vi "test_riccat_02i.vi"() -> (3 "All Tests Passed":bool)   [LabVIEW 2019]
uses:
  <vilib>/Analysis/Matrix/Datatypes/RealMatrix.ctl
  <vilib>/Analysis/7linalg.llb/Real Transpose Matrix.vi
  <vilib>/Analysis/baseanly.llb/Real A x B.vi
  <vilib>/Analysis/Matrix/Numeric/Subtract/Subtract - RM,RM.vi
  <vilib>/Analysis/Matrix/Numeric/Add/Add - RM,RM.vi
  <vilib>/Analysis/baseanly.llb/Real Inverse Matrix.vi
  <vilib>/Analysis/Matrix/Numeric/Absolute Value/Absolute Value - RM.vi
  <vilib>/Rock Robotics/WPI/ThirdParty/JAS_Junk/TrajLib/Trajectory_Library.lvlib
  <vilib>/Analysis/NI_AALPro.lvlib
  <vilib>/Analysis/NI_AALBase.lvlib
  <vilib>/Analysis/Matrix/NI_Matrix.lvlib
panel:
  out "Error":bool
  out "Iterations":i32
  out "Elapsed \nTime MS":dbl
  out "Err 4":i32
  out "Err 3":i32
  out "Err 2":i32
  out "Err 1":i32
  out "Err 9":i32
  out "ZERO":T1
  out "X  Answer":T1
  in  "R":T1=[[0.3]]
  in  "Q":T1=[[1.0, 0.0], [0.0, 0.0]]
  in  "B":T1=[[0.0], [1.0]]
  in  "A":T1=[[1.0, 1.0], [0.0, 1.0]]
  # "// ------------------------------------------------------------\n  // Test 2: invertible A"
  # "A2 << \n             1, 1, \n              0, 1;"
  # "B2 << \n        0, \n        1;"
  # "Solution weight ??"
  # "Q2 << \n         1, 0, \n         0, 0;"
  # "Example G2"
  # "Cost ??"
  # "R2 << 0.3;"
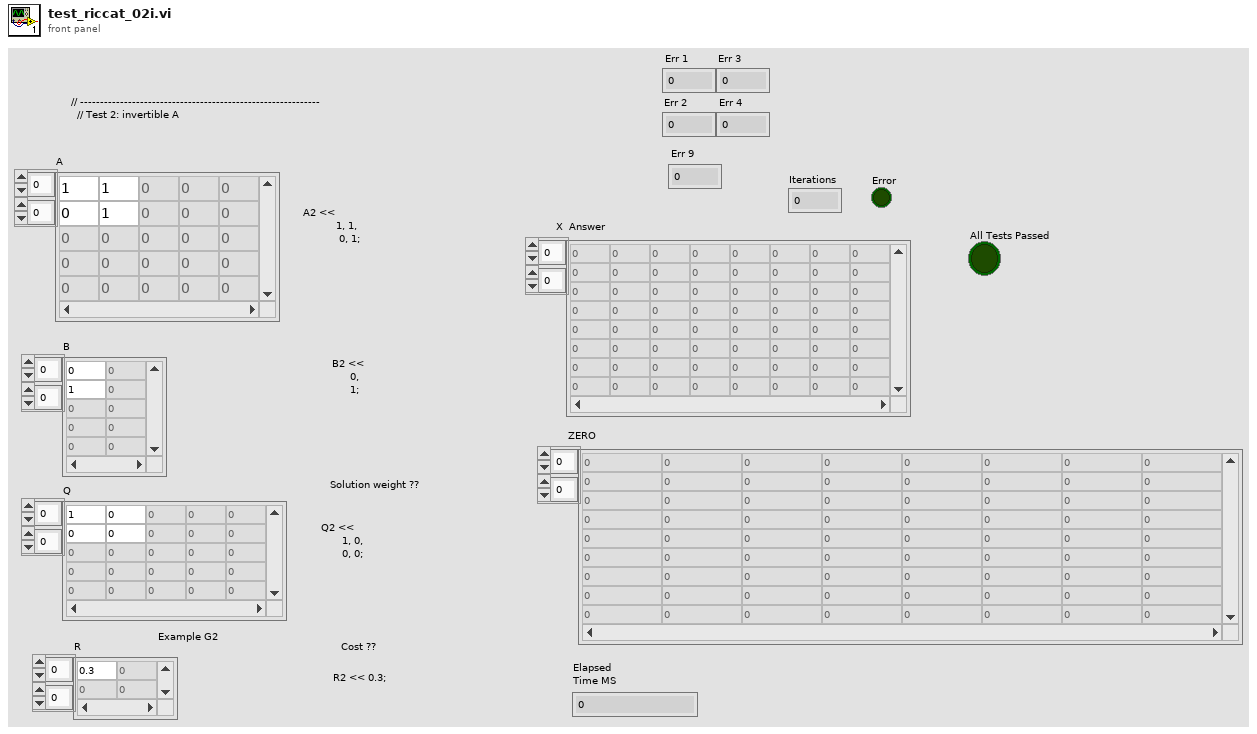
[diagram p1: front panel]
types:
  T1 = typedef "NI_Matrix.lvlib/RealMatrix.ctl" = dbl[][]
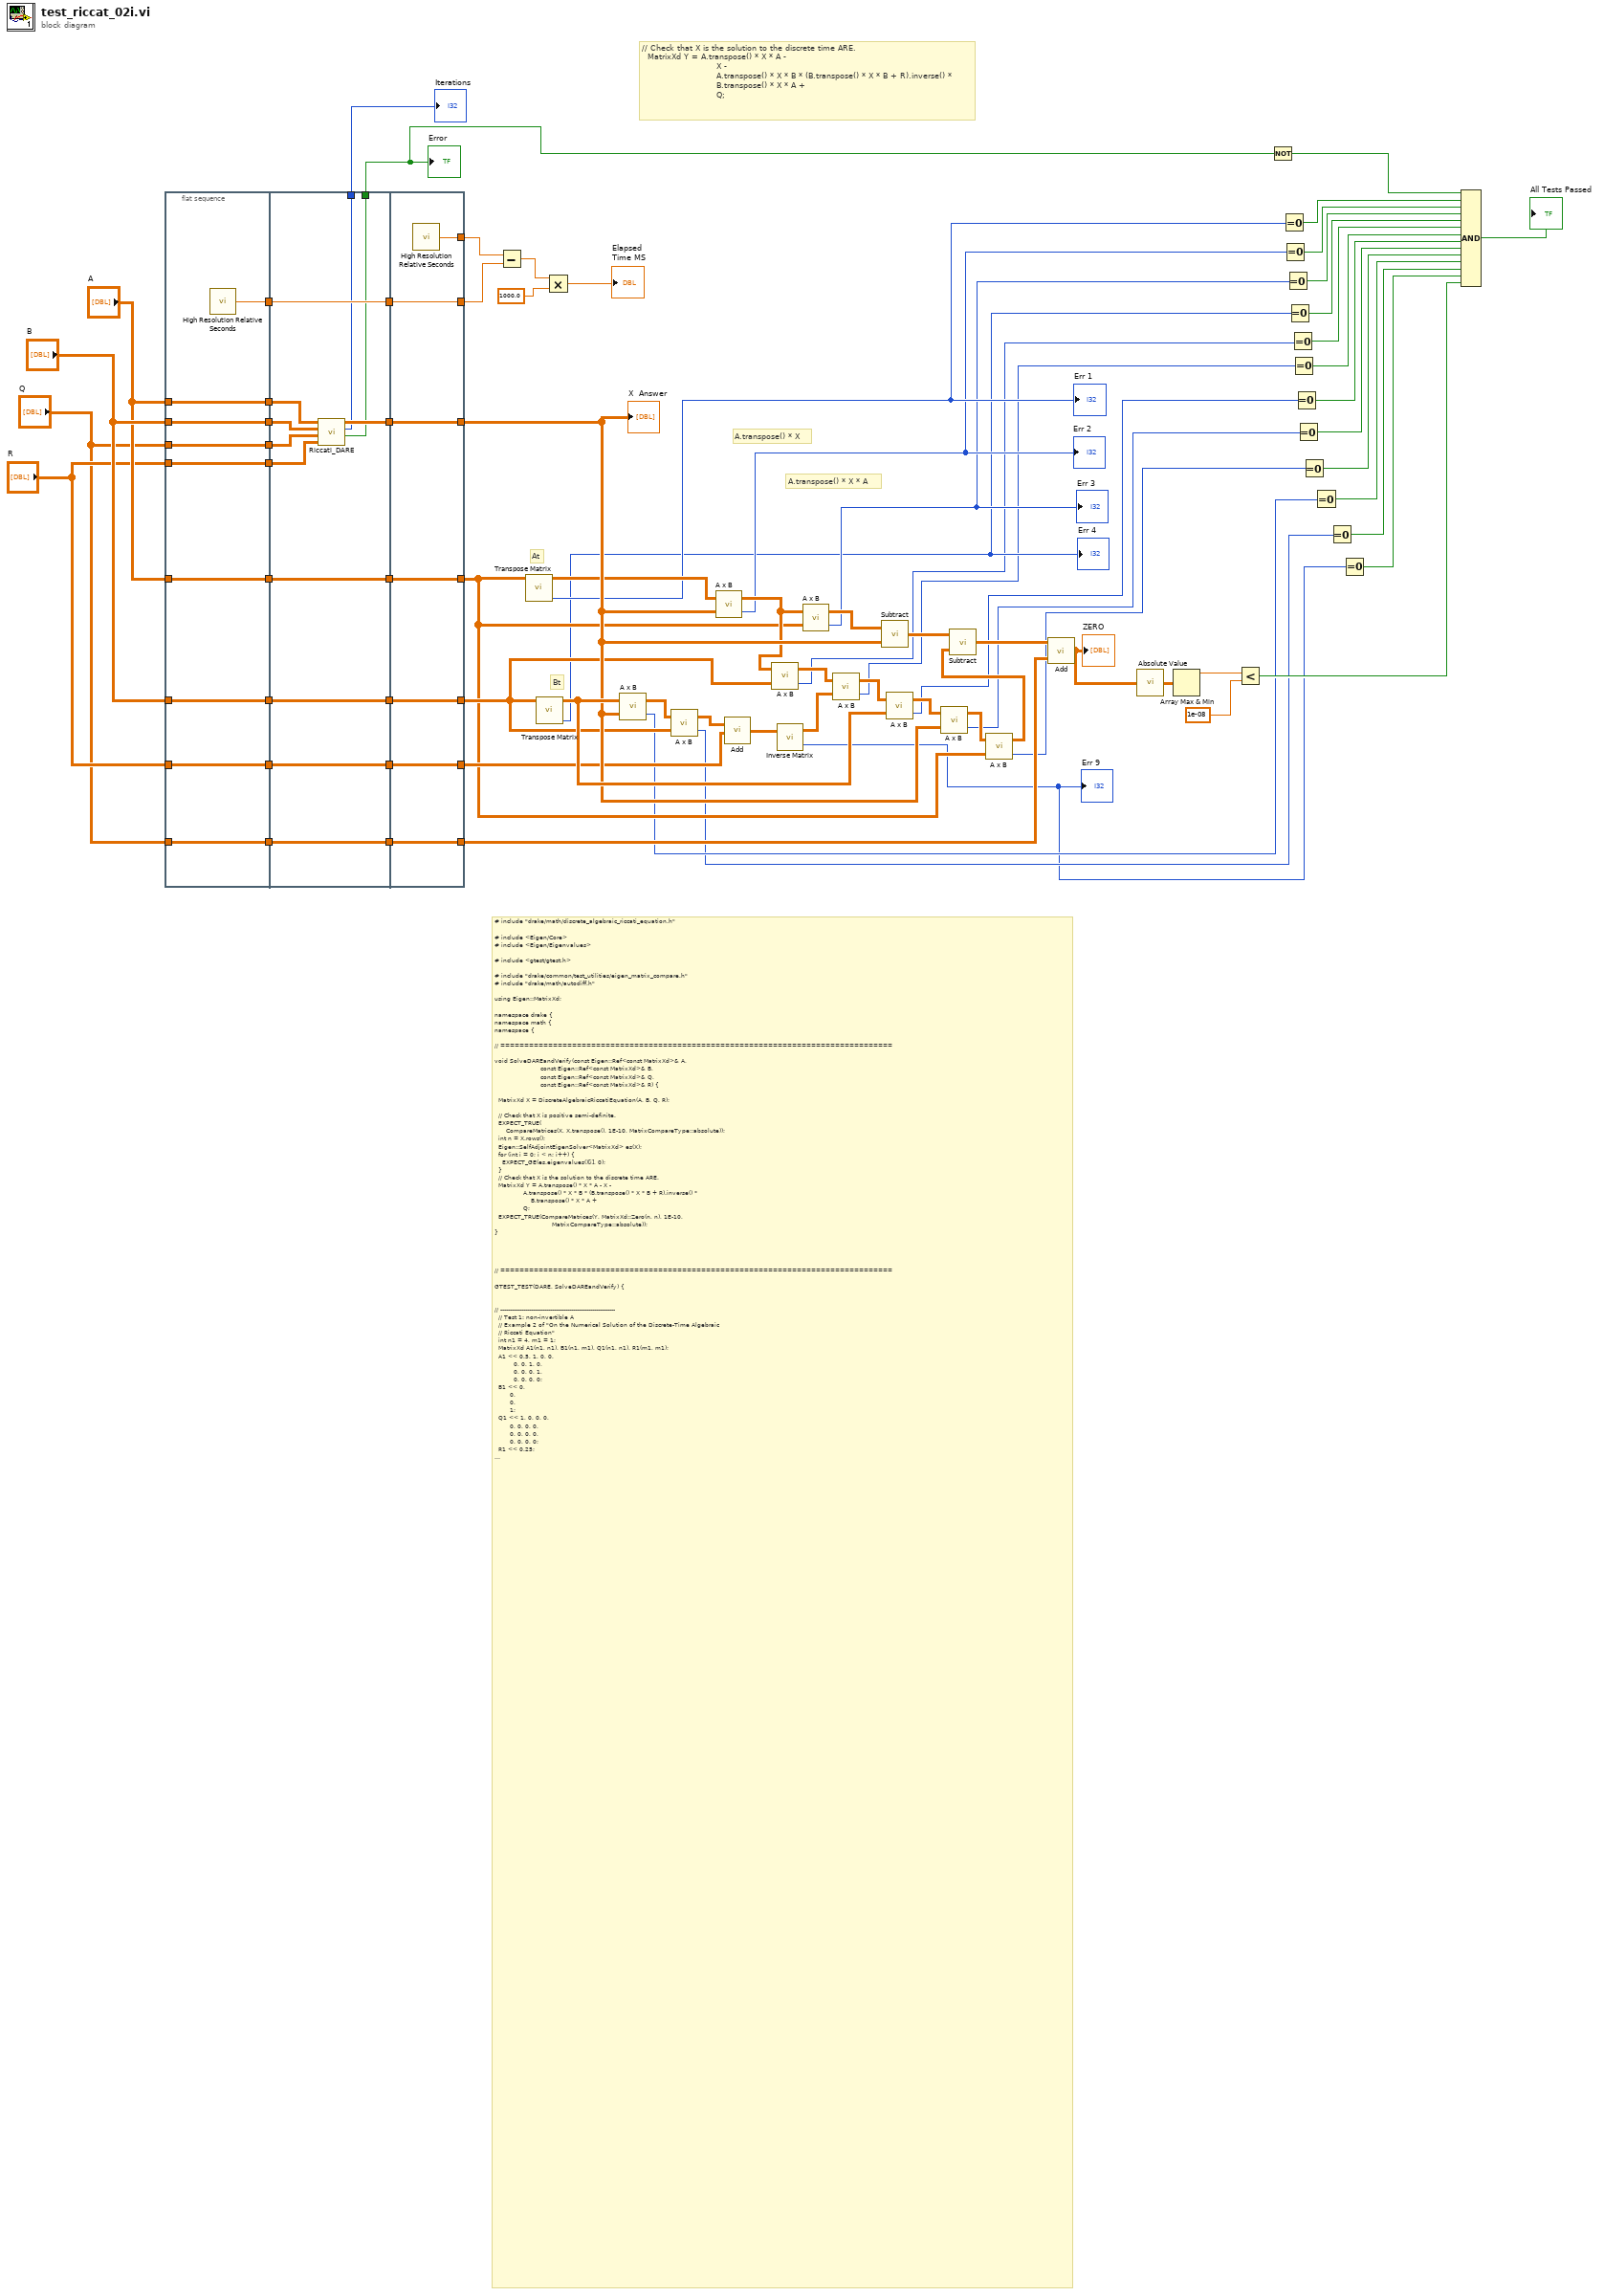
[diagram p0: block diagram]
diagram:
  # "A.transpose() * X"
  # "A.transpose() * X * A"
  # "Bt"
  # "At"
  # "// Check that X is the solution to the discrete time ARE.\n  MatrixXd Y = A.transpose() * X * A - \n                          X -\n                          A.transpose() * X * B * (B.transpose() * X * B + R).inverse() *\n                          B.transpose() * X * A +\n                          Q;"
  # "# include \"drake/math/discrete_algebraic_riccati_equation.h\"\n\n# include <Eigen/Core>\n# include <Eigen/Eigenvalues>\n\n# include <gtest/gtest.h>\n\n# include \"drake/common/test_utilities/eigen_matrix_compare.h\"\n# include \"drake/math/autodiff.h\"\n\nusing Eigen::MatrixXd;\n\nnamespace drake {\nnamespace math {\nnamespace {\n\n// ==================================================================================\n\nvoid SolveDAREandVerify(const Eigen::Ref<const MatrixXd>& A,\n                        const Eigen::Ref<const MatrixXd>& B,\n                        const Eigen::Ref<const MatrixXd>& Q,\n                        const Eigen::Ref<const MatrixXd>& R) {\n\n  MatrixXd X = DiscreteAlgebraicRiccatiEquation(A, B, Q, R);\n\n  // Check that X is positive semi-definite.\n  EXPECT_TRUE(\n      CompareMatrices(X, X.transpose(), 1E-10, MatrixCompareType::absolute));\n  int n = X.rows();\n  Eigen::SelfAdjointEigenSolver<MatrixXd> es(X);\n  for (int i = 0; i < n; i++) {\n    EXPECT_GE(es.eigenvalues()[i], 0);\n  }\n  // Check that X is the solution to the discrete time ARE.\n  MatrixXd Y = A.transpose() * X * A - X -\n               A.transpose() * X * B * (B.transpose() * X * B + R).inverse() *\n                   B.transpose() * X * A +\n               Q;\n  EXPECT_TRUE(CompareMatrices(Y, MatrixXd::Zero(n, n), 1E-10,\n                              MatrixCompareType::absolute));\n}\n\n\n\n\n// ==================================================================================\n\nGTEST_TEST(DARE, SolveDAREandVerify) {\n\n\n// ------------------------------------------------------------\n  // Test 1: non-invertible A\n  // Example 2 of \"On the Numerical Solution of the Discrete-Time Algebraic\n  // Riccati Equation\"\n  int n1 = 4, m1 = 1;\n  MatrixXd A1(n1, n1), B1(n1, m1), Q1(n1, n1), R1(m1, m1);\n  A1 << 0.5, 1, 0, 0, \n          0, 0, 1, 0, \n          0, 0, 0, 1, \n          0, 0, 0, 0;\n  B1 << 0, \n        0, \n        0, \n        1;\n  Q1 << 1, 0, 0, 0, \n        0, 0, 0, 0, \n        0, 0, 0, 0, \n        0, 0, 0, 0;\n  R1 << 0.25;\n  SolveDAREandVerify(A1, B1, Q1, R1);\n// ------------------------------------------------------------\n  // Test 2: invertible A\n  int n2 = 2, m2 = 1;\n  MatrixXd A2(n2, n2), B2(n2, m2), Q2(n2, n2), R2(m2, m2);\n  A2 << 1, 1, 0, 1;\n  B2 << 0, 1;\n  Q2 << 1, 0, 0, 0;\n  R2 << 0.3;\n  SolveDAREandVerify(A2, B2, Q2, R2);\n\n// ------------------------------------------------------------\n  // Test 3: the first generalized eigenvalue of (S,T) is stable\n  int n3 = 2, m3 = 1;\n  MatrixXd A3(n3, n3), B3(n3, m3), Q3(n3, n3), R3(m3, m3);\n  A3 << 0, 1, 0, 0;\n  B3 << 0, 1;\n  Q3 << 1, 0, 0, 1;\n  R3 << 1;\n  SolveDAREandVerify(A3, B3, Q3, R3);\n\n// ------------------------------------------------------------\n  // Test 4: A = B = Q = R = I_2 (2-by-2 identity matrix)\n  int n4 = 2, m4 = 2;\n  MatrixXd A4(n4, n4), B4(n4, m4), Q4(n4, n4), R4(m4, m4);\n  A4 << 1, 0, 0, 1;\n  B4 << 1, 0, 0, 1;\n  Q4 << 1, 0, 0, 1;\n  R4 << 1, 0, 0, 1;\n  SolveDAREandVerify(A4, B4, Q4, R4);\n\n// ------------------------------------------------------------\n}\n}  // namespace\n}  // namespace math\n}  // namespace drake"
  n1 = flat-sequence {
    tunnel: "B" -> [w81]
    tunnel: "A" -> [w82]
    tunnel: "B" -> [w83]
    tunnel: "Q" -> [w84]
    tunnel: "A" -> [w85]
    tunnel: "R" -> [w86]
    tunnel: [w86] -> w61
    tunnel: [w85] -> w60
    tunnel: [w84] -> w59
    tunnel: [w83] -> w58
    tunnel: [w82] -> w57
    tunnel: [w81] -> w56
    tunnel: "R" -> [w80]
    tunnel: [w80] -> w48
    tunnel: "Q" -> [w79]
    tunnel: [w79] -> w45
    tunnel: [w78] -> w38
    tunnel: w61 -> [w98]
    tunnel: w60 -> [w96]
    tunnel: w59 -> [w95]
    tunnel: w58 -> [w94]
    tunnel: w57 -> [w93]
    tunnel: w56 -> [w92]
    tunnel: [w97] -> w55
    tunnel: [w93] -> w54
    tunnel: [w92] -> w53
    tunnel: [w91] -> w49
    tunnel: w48 -> [w91]
    tunnel: w45 -> [w90]
    tunnel: [w90] -> w44
    tunnel: [w89] -> w39
    tunnel: w38 -> [w89]
    tunnel: [w88] -> w34
    tunnel: [w87] -> w18
    tunnel: [w103] -> w51
    tunnel: [w104] -> w33
    tunnel: [w105] -> w69
    tunnel: w55 -> [w105]
    tunnel: w54 -> [w104]
    tunnel: w53 -> [w103]
    tunnel: [w102] -> w46
    tunnel: w49 -> [w102]
    tunnel: [w101] -> w42
    tunnel: w44 -> [w101]
    tunnel: [w100] -> w41
    tunnel: [w99] -> w40
    tunnel: w39 -> [w99]
    frame #0 {
      n2 = call <vilib>:"High Resolution Relative Seconds.vi"() -> ("relative seconds"=w78:dbl)
    }
    frame #1 {
      n3 = call <vilib>:"Riccati_DARE.vi"("R"=w98, "Q"=w95, "B"=w94, "A"=w96) -> ("Error"=w87:bool, "Iterations"=w88:i32, "Answer"=w97:T1)  [unwired: 5 in]
    }
    frame #2 {
      n4 = call <vilib>:"High Resolution Relative Seconds.vi"() -> ("relative seconds"=w100:dbl)
    }
  }
  n5 = Subtract(x=w41, y=w40) -> (x-y=w37:dbl)
  n6 = call-poly <vilib>:"Transpose Matrix.vi"("Input Matrix"=w33) -> ("error"=w17:i32, "Matrix Transpose"=w62:T1)  [unwired: 9 in]
  "Err 1" <- w17
  n7 = call-poly <vilib>:"Transpose Matrix.vi"("Input Matrix"=w51) -> ("error"=w14:i32, "Matrix Transpose"=w71:T1)  [unwired: 9 in]
  "Err 4" <- w14
  n8 = Multiply(x=w37, y=1000.0) -> (x*y=→"Elapsed \nTime MS":dbl)
  n9 = call-poly <vilib>:"A x B.vi"("B"=w69, "A"=w71) -> ("error"=w3:i32, "A x B"=w76:T1)
  n10 = call-poly <vilib>:"A x B.vi"("B"=w51, "A"=w76) -> ("error"=w2:i32, "A x B"=w75:T1)
  n11 = call-poly <vilib>:"A x B.vi"("B"=w69, "A"=w62) -> ("error"=w16:i32, "A x B"=w64:T1)
  "Err 2" <- w16
  n12 = call-poly <vilib>:"Add.vi"("Real Matrix B"=w46, "Real Matrix A"=w75) -> ("A + B"=w74:T1)
  n13 = call-poly <vilib>:"A x B.vi"("B"=w51, "A"=w64) -> ("error"=w8:i32, "A x B"=w63:T1)
  n14 = call-poly <vilib>:"Inverse Matrix.vi"("Input Matrix"=w74) -> ("error"=w1:i32, "Inverse Matrix"=w73:T1)  [unwired: 1 in]
  "Err 9" <- w1
  n15 = call-poly <vilib>:"A x B.vi"("B"=w33, "A"=w64) -> ("error"=w15:i32, "A x B"=w77:T1)
  "Err 3" <- w15
  n16 = call-poly <vilib>:"A x B.vi"("B"=w73, "A"=w63) -> ("error"=w7:i32, "A x B"=w72:T1)
  n17 = call-poly <vilib>:"Subtract.vi"("Real Matrix B"=w69, "Real Matrix A"=w77) -> ("A - B"=w67:T1)
  n18 = call-poly <vilib>:"A x B.vi"("B"=w71, "A"=w72) -> ("error"=w6:i32, "A x B"=w70:T1)
  n19 = call-poly <vilib>:"A x B.vi"("B"=w69, "A"=w70) -> ("error"=w5:i32, "A x B"=w68:T1)
  n20 = call-poly <vilib>:"A x B.vi"("B"=w33, "A"=w68) -> ("error"=w4:i32, "A x B"=w66:T1)
  n21 = call-poly <vilib>:"Subtract.vi"("Real Matrix B"=w66, "Real Matrix A"=w67) -> ("A - B"=w65:T1)
  n22 = call-poly <vilib>:"Add.vi"("Real Matrix B"=w42, "Real Matrix A"=w65) -> ("A + B"=w13:T1)
  "ZERO" <- w13
  n23 = call-poly <vilib>:"Absolute Value.vi"("Real Matrix A"=w13) -> ("|A|"=w12:T1)
  n24 = Array Max & Min(array=w12) -> (max value=w11:dbl)  [unwired: 3 out]
  n25 = Less?(x=w11, y=1e-08) -> (x < y?=w9:bool)
  n26 = Not(x=w18) -> (.not. x?=w19:bool)
  n27 = Equal To 0?(x=w17) -> (x = 0?=w31:bool)
  n28 = Equal To 0?(x=w16) -> (x = 0?=w30:bool)
  n29 = Equal To 0?(x=w15) -> (x = 0?=w29:bool)
  n30 = Equal To 0?(x=w14) -> (x = 0?=w28:bool)
  n31 = Equal To 0?(x=w8) -> (x = 0?=w27:bool)
  n32 = Equal To 0?(x=w7) -> (x = 0?=w26:bool)
  n33 = Equal To 0?(x=w6) -> (x = 0?=w25:bool)
  n34 = Equal To 0?(x=w5) -> (x = 0?=w24:bool)
  n35 = Equal To 0?(x=w4) -> (x = 0?=w23:bool)
  n36 = Equal To 0?(x=w3) -> (x = 0?=w22:bool)
  n37 = Equal To 0?(x=w2) -> (x = 0?=w21:bool)
  n38 = Equal To 0?(x=w1) -> (x = 0?=w20:bool)
  n39 = Compound Arithmetic op=AND(w19, w31, w30, w29, w28, w27, w26, w25, w24, w23, w22, w21, w20, w9) -> (→"All Tests Passed":bool)
  "X  Answer" <- w69
  "Iterations" <- w34
  "Error" <- w18
